vi "example-InsertMenubarItem.vi"() -> ()   [LabVIEW 2020]
uses:
  a1b5153a-e3ee-49e1-af71-bc127d6ac68d.vi
panel:
  in  "String":string
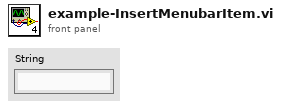
[diagram p1: front panel]
types:
  T1 = cluster{"Name":string, "Include Shift Key?":bool, "Include Ctrl Key?":bool, "Shortcut Key":string}[]
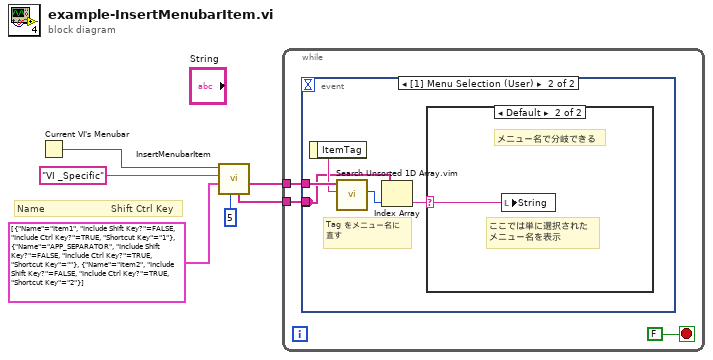
[diagram p0: block diagram]
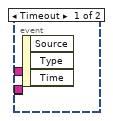
[diagram p2: hidden frame]
diagram:
  # "Name                      Shift Ctrl Key"
  n1 = Current VI's Menubar() -> (w6:refnum<k9>)
  n2 = call "InsertMenubarItem.vi"("Insert After (last)"=5, "Sub Items"=T1 [{"Name"="Item1", "Include Shift Key?"=FALSE, "Include Ctrl Key?"=TRUE, "Shortcut Key"="1"}, {"Name"="APP_SEPARATOR", "Include Shift Key?"=FALSE, "Include Ctrl Key?"=TRUE, "Shortcut Key"=""}, {"Name"="Item2", "Include Shift Key?"=FALSE, "Include Ctrl Key?"=TRUE, "Shortcut Key"="2"}], "Menu Name"="VI _Specific", "menu ref"=w6) -> ("Sub Item Tags"=w2:string[], "Sub Item Names"=w1:string[])  [unwired: 3 in, 3 out]
  n3 = while {
    tunnel: w2 -> [w8]
    tunnel: w1 -> [w7]
    stop <- FALSE stop-if-true
    n4 = event shown="[1] Menu Selection (User)" {
      selector: _ -> [_ _]
      dyn-events: _ -> [_ _]
      timeout: _ -> [_ _]
      tunnel: w8 -> [_ w14]
      tunnel: [_ w12] -> _
      tunnel: w7 -> [_ w12]
      event Timeout {
        n5 = event-data() -> ()  [unwired: 1 in, 3 out]
      }
      event Menu Selection (User) {
        # "Tag をメニュー名に\n直す"
        n6 = event-data() -> ("ItemTag"=w13:string)  [unwired: 1 in]
        n7 = call "Search Unsorted 1D Array.vim"("element"=w13, "unsorted 1D array"=w14) -> ("index of element"=w11:i32)  [unwired: 9 in]
        n8 = Index Array(array=w12, index=w11) -> (element=w10:string)
        n9 = case shown="Default" w10 {
          selector: w10 -> [_ w15]
          frame "" {
          }
          frame Default {
            # "ここでは単に選択された\nメニュー名を表示"
            # "メニュー名で分岐できる"
            n10 = local write "String"(w15) -> ()
          }
        }
      }
    }
  }
